vi "set task token.vi"(10 "task token":refnum<class "null task token.lvclass">, 11 "task in":refnum<class "task.lvclass">) -> (3 "task out":refnum<class "task.lvclass">)   [LabVIEW 2013, in "task.lvclass"]
uses:
  task.lvclass
  task token/null task token.lvclass
  task.lvclass/task.ctl
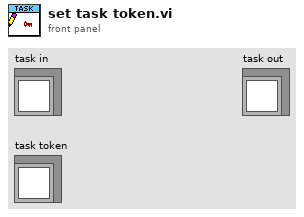
[diagram p1: front panel]
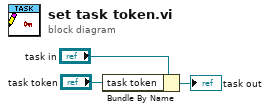
[diagram p0: block diagram]
diagram:
  n1 = Bundle By Name(cluster="task in", "task token"="task token") -> (→"task out":refnum<class "task.lvclass">)
